vi "PFY.vi"(8 "错误输入":errorcluster) -> (0 "错误输出":errorcluster, 3 "输出簇":cluster{"PASS":u32, "Total":u32, "Rate":dbl})   [LabVIEW 2013]
uses:
  Global constant.vi
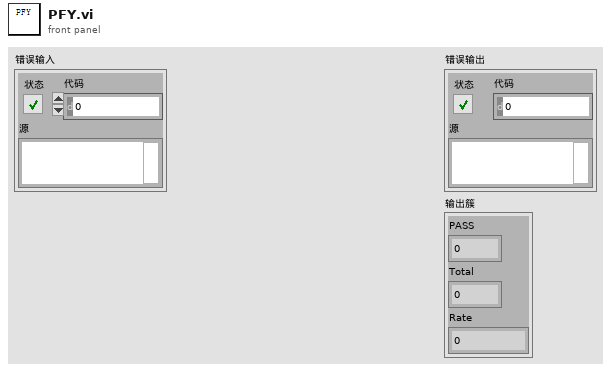
[diagram p1: front panel]
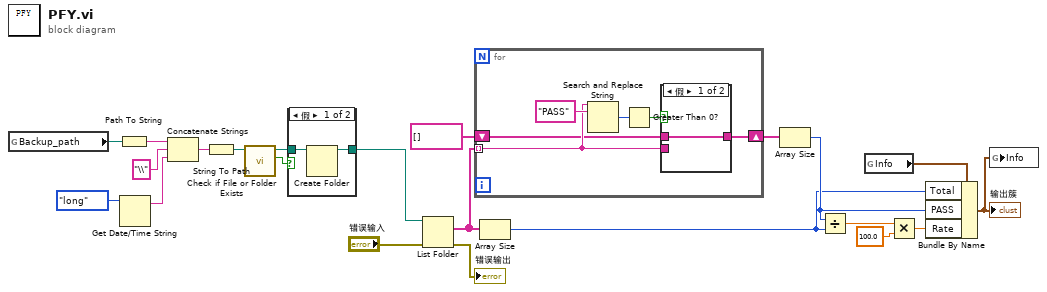
[diagram p0: block diagram]
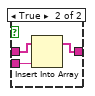
[diagram p3: hidden frame]
diagram:
  n1 = global read "Global constant.vi" "Backup_path"() -> (w17:path)
  n2 = Path To String(path=w17) -> (string=w18:string)
  n3 = Get Date/Time String(date format (0)=enum16{"short", "long", "abbreviated"}."long") -> (date string=w20:string)  [unwired: 2 in, 1 out]
  n4 = Concatenate Strings(w18, "\\", w20) -> (w19:string)
  n5 = String To Path(string=w19) -> (path=w4:path)
  n6 = call <vilib>:"Check if File or Folder Exists.vi"("path"=w4) -> ("file or folder exists?"=w3:bool, "dup path"=w2:path)  [unwired: 8 in, 1 out]
  n7 = case shown="假" w3 {
    tunnel: w2 -> [w24 w25]
    tunnel: [w23 w25] -> w1
    frame False {
      n8 = Create Folder(path (use dialog)=w24) -> (created path=w23:path)  [unwired: 2 in, 2 out]
    }
    frame True {
    }
  }
  n9 = List Folder(path=w1, error in="错误输入") -> (filenames=w14:string[], error out=→"错误输出":errorcluster)  [unwired: 2 in, 2 out]
  n10 = for {
    tunnel: w14 -> [w28] mode=indexing
    shift-right: [w27] -> w12
    shift-left: string[] [] -> [w26]
    n11 = Search and Replace String(input string=w28, search string="PASS" ("搜索字符串")) -> (number of replacements=w30:i32)  [unwired: 6 in, 3 out]
    n12 = Greater Than 0?(x=w30) -> (x > 0?=w29:bool)
    n13 = case shown="假" w29 {
      tunnel: w28 -> [_ w35]
      tunnel: [w32 w34] -> w27
      tunnel: w26 -> [w32 w33]
      frame False {
      }
      frame True {
        n14 = Insert Into Array(array=w33, new element=w35) -> (w34:string[])  [unwired: 1 in]
      }
    }
  }
  n15 = Array Size(array=w14) -> (size(s)=w10:i32)
  n16 = Array Size(array=w12) -> (size(s)=w11:i32)
  n17 = Divide(x=w11, y=w10) -> (x/y=w9:dbl)
  n18 = global read "Global constant.vi" "Info"() -> (w16:cluster{"PASS":u32, "Total":u32, "Rate":dbl})
  n19 = Multiply(x=w9, y=100.0) -> (x*y=w7:dbl)
  n20 = Bundle By Name(cluster=w16, "Total"=w10, "PASS"=w11, "Rate"=w7) -> (w15:cluster{"PASS":u32, "Total":u32, "Rate":dbl})
  "输出簇" <- w15
  n21 = global write "Global constant.vi" "Info"(w15) -> ()
